vi "create.vi"(8 "error in":errorcluster, 11 "API Token (string or path)":string) -> (0 "error out":errorcluster, 3 "Nominal Client":refnum<class "Nominal Client.lvclass">)   [LabVIEW 2018, in "Nominal Client.lvclass"]
doc: "Click on <b>Detailed help</b> to get your API Token from your nominal account.\n\nConnect to the API using your API token.\n1) Create a text file that contains your API token.\n2) Wire a string containing your API token directly.\n3) For development, wire an empty string. When an empty string is wired, the API will look for a `.token` file in your application's directory.\n\nNOTE: Besure to exclude API Tokens (and token files) from source code control."
uses:
  Nominal Client.lvclass
  <vilib>/addons/_JKI.lib/REST Client/classes/REST Client/REST Client.lvclass
  private_data.ctl
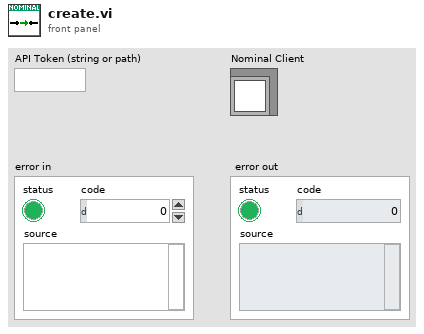
[diagram p1: front panel]
types:
  T1 = typedef "Nominal Client.lvclass/private_data.ctl" = cluster{"API Token":string, "REST Client":refnum<class "REST Client.lvclass">}
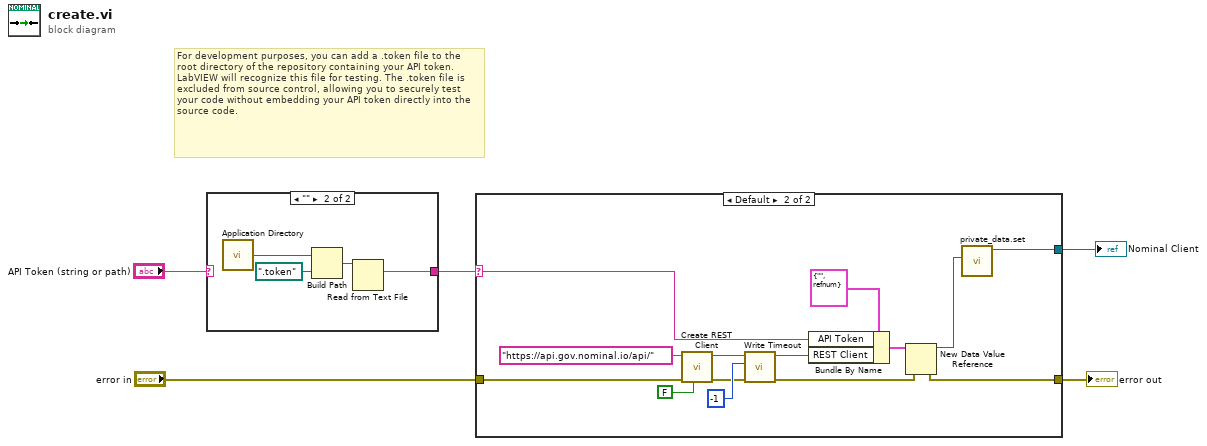
[diagram p0: block diagram]
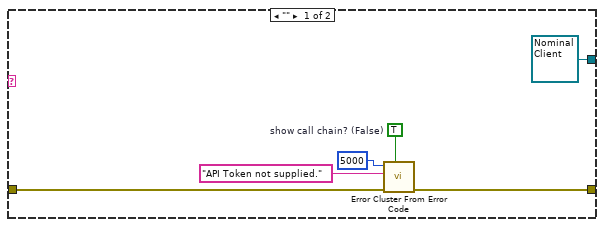
[diagram p3: hidden frame]
diagram:
  # "For development purposes, you can add a .token file to the root directory of the repository containing your API token. LabVIEW will recognize this file for testing. The .token file is excluded from source control, allowing you to securely test your code without embedding your API token directly into the source code."
  n1 = case shown="\"\"" "API Token (string or path)" {
    selector: "API Token (string or path)" -> [w6 _]
    tunnel: [w6 w7] -> w2
    frame Default {
    }
    frame "" {
      n2 = call <vilib>:"Application Directory.vi"() -> ("Application Directory"=w10:path)
      n3 = Build Path(base path=w10, name or relative path=path ".token") -> (appended path=w8:path)
      n4 = Read from Text File(file (use dialog)=w8) -> (text=w7:string)  [unwired: 3 in, 3 out]
    }
  }
  n5 = case shown="Default" w2 {
    selector: w2 -> [_ w24]
    tunnel: "error in" -> [w12 w26]
    tunnel: [refnum<class "Nominal Client.lvclass"> refnum ("Nominal Client") w22] -> w5
    tunnel: [w11 w25] -> w4
    frame "" {
      w13 = TRUE  # show call chain? (False)
      n6 = call <vilib>:"Error Cluster From Error Code.vi"("show call chain? (False)"=w13, "error in (no error)"=w12, "error message (\"\")"="API Token not supplied." ("error message (\"\")"), "error code (0)"=5000) -> ("error out"=w11:errorcluster)  [unwired: 5 in]
    }
    frame Default {
      n7 = call <vilib>:"Create REST Client.vi"("Verify Server(true)"=FALSE, "error in (no error)"=w26, "Base URL"="https://api.gov.nominal.io/api/") -> ("error out"=w19:errorcluster, "REST Client out"=w20:refnum<class "REST Client.lvclass">)  [unwired: 7 in]
      n8 = call-dynamic "Write Timeout.vi"("error in (no error)"=w19, "Timeout"=-1, "REST Client in"=w20) -> ("error out"=w18:errorcluster, "REST Client out"=w17:refnum<class "REST Client.lvclass">)  [unwired: 7 in]
      n9 = Bundle By Name(cluster=T1 {"API Token"="", "REST Client"=refnum} ("Cluster of class private data"), "API Token"=w24, "REST Client"=w17) -> (w29:T1)
      n10 = New Data Value Reference(data value=w29, error in=w18) -> (data value reference=w23:refnum<data-value>, error out=w25:errorcluster)
      n11 = call "private_data.set.vi"("private data"=w23) -> ("Nominal Client"=w22:refnum<class "Nominal Client.lvclass">)  [unwired: 10 in]
    }
  }
  "Nominal Client" <- w5
  "error out" <- w4
